vi "Counter.vi"(8 "error in (no error)":errorcluster, 11 "Reset(T)/Count(F)":bool) -> (0 "error out":errorcluster, 3 "Counter":u32)   [LabVIEW 2020]
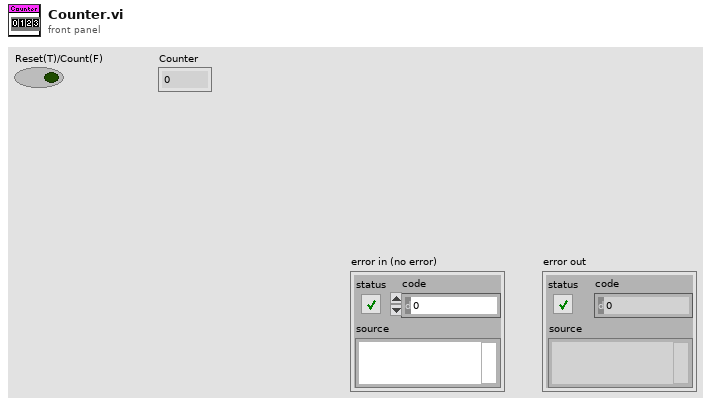
[diagram p1: front panel]
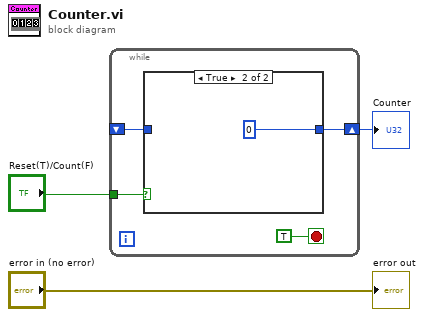
[diagram p0: block diagram]
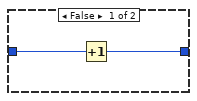
[diagram p2: hidden frame]
diagram:
  n1 = while {
    tunnel: "Reset(T)/Count(F)" -> [w6]
    shift-right: [w5] -> w3
    shift-left: _ -> [w4]
    stop <- TRUE stop-if-true
    n2 = case shown="True" w6 {
      tunnel: [w8 u32 0 ("Counter")] -> w5
      tunnel: w4 -> [w9 _]
      frame False {
        n3 = Increment(x=w9) -> (x+1=w8:u32)
      }
      frame True {
      }
    }
  }
  "Counter" <- w3
  "error out" <- "error in (no error)"
